vi "MetaDataToCenterFastSlow.vi"(2 "Galvo.center":cluster{dbl, dbl}, 3 "MetaData":string, 4 "ScanRotation":dbl) -> (0 "Fast/Slow":cluster{dbl, dbl}[](array[cluster]), 1 "Center":cluster{dbl, dbl})   [LabVIEW 2011]
panel:
  out "CenterOfImageInScanKoordiantes":cluster{"meter":dbl, "meter":dbl}
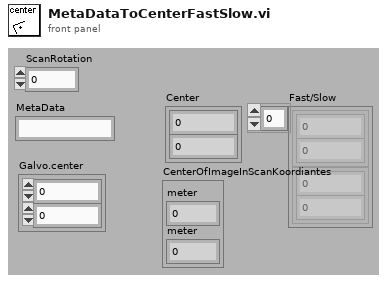
[diagram p1: front panel]
types:
  T1 = typedef "ScanControl.ctl" = cluster{"Time [s]":dbl, "action":T2, "channel":T3, "value (/s)":dbl}[]
  T2 = typedef "ScanControl_Action.ctl" = enum16{"Abs", "Rel", "Inc", "IncInc", "LoopStart", "LoopEnd", "WaitTriggerRising"}
  T3 = typedef "ScanControl_Channel.ctl" = enum16{"Com", "AnalogConfig", "AnalogValue", "GalvoX", "GalvoY", "Galvo3", "Galvo4", "Digital", "Free", "Loop", "SMoveTime", "Image1X", "Image1Y", "Image2X", "Image2Y"}
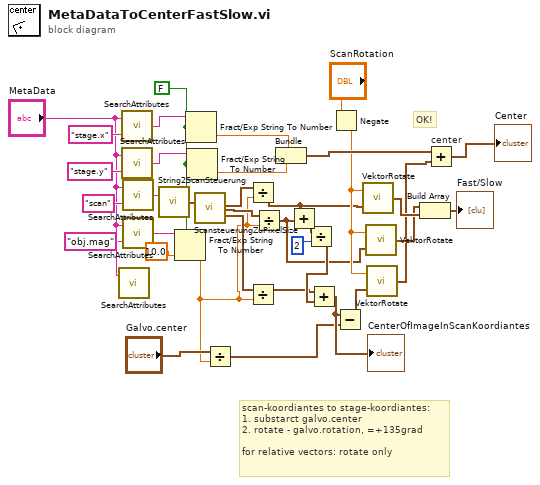
[diagram p0: block diagram]
diagram:
  w7 = FALSE ("Systemdezimalzeichen verwenden (T)")
  # "scan-koordiantes to stage-koordiantes:\n1. substarct galvo.center\n2. rotate - galvo.rotation, =+135grad\n\nfor relative vectors: rotate only"
  # "OK!"
  n1 = call "SearchAttributes.vi"("String"="MetaData") -> ()  [unwired: 1 in, 1 out]
  n2 = call "SearchAttributes.vi"("Search"="stage.x", "String"="MetaData") -> ("ValueText"=w20:string)
  n3 = call "SearchAttributes.vi"("Search"="stage.y", "String"="MetaData") -> ("ValueText"=w21:string)
  n4 = call "SearchAttributes.vi"("Search"="scan", "String"="MetaData") -> ("ValueText"=w23:string)
  n5 = call "SearchAttributes.vi"("Search"="obj.mag", "String"="MetaData") -> ("ValueText"=w9:string)
  n6 = call "String2ScanSteuerung.vi"("String"=w23) -> ("ScanSteuerung"=w24:T1)
  n7 = Fract/Exp String To Number(use system decimal point (T)=w7, string=w9, default (0 dbl)=10.0 ("Standard (0 DBL)")) -> (number=w1:dbl)  [unwired: 2 out]
  n8 = Fract/Exp String To Number(use system decimal point (T)=w7, string=w20) -> (number=w25:dbl)  [unwired: 3 out]
  n9 = Fract/Exp String To Number(use system decimal point (T)=w7, string=w21) -> (number=w26:dbl)  [unwired: 3 out]
  n10 = call "ScansteuerungZuPixelSize.vi"("ScanSteuerung"=w24) -> ("Slow-Vektors"=w14:cluster{"meter":dbl, "meter":dbl}, "last-fast-vektor (exact)"=w2:cluster{"meter":dbl, "meter":dbl}, "xyStart"=w33:cluster{"meter":dbl, "meter":dbl})  [unwired: 1 in, 15 out]
  n11 = Divide(x="Galvo.center", y=w1) -> (x/y=w6:cluster{dbl, dbl})
  n12 = Divide(x=w14, y=w1) -> (x/y=w5:cluster{"meter":dbl, "meter":dbl})
  n13 = Divide(x=w33, y=w1) -> (x/y=w3:cluster{"meter":dbl, "meter":dbl})
  n14 = Divide(x=w2, y=w1) -> (x/y=w4:cluster{"meter":dbl, "meter":dbl})
  n15 = Bundle(w25, w26) -> (w31:cluster{dbl, dbl})  [unwired: 1 out]
  n16 = Add(x=w5, y=w4) -> (x+y=w34:cluster{"meter":dbl, "meter":dbl})
  n17 = Divide(x=w34, y=2) -> (x/y=w36:cluster{"meter":dbl, "meter":dbl})
  n18 = Add(x=w3, y=w36) -> (x+y=w12:cluster{"meter":dbl, "meter":dbl})
  "CenterOfImageInScanKoordiantes" <- w12
  n19 = Negate(x="ScanRotation") -> (-x=w15:dbl)
  n20 = Subtract(x=w12, y=w6) -> (x-y=w11:cluster{dbl, dbl})
  n21 = call "VektorRotate.vi"("xyStart"=w5, "angel [rad]"=w15) -> ("rotated point"=w29:cluster{dbl, dbl})
  n22 = call "VektorRotate.vi"("xyStart"=w4, "angel [rad]"=w15) -> ("rotated point"=w28:cluster{dbl, dbl})
  n23 = call "VektorRotate.vi"("xyStart"=w11, "angel [rad]"=w15) -> ("rotated point"=w13:cluster{dbl, dbl})
  n24 = Build Array(w28, w29) -> (→"Fast/Slow":cluster{dbl, dbl}[])
  n25 = Add "center"(x=w31, y=w13) -> (x+y=→"Center":cluster{dbl, dbl})
